vi "FGVScanParametersWaveform.vi"(7 "Enum":T3, 8 "error in":errorcluster, 9 "Parameters In":T1={"fastRoundPts"=32, "slowRoundPts"=8, "fastWaveType"=enum."Rounded", "slowWaveType"=enum."Triangle", "fastWavePts"=1024, "slowWavePts"=1024, "outputRateHz"=800000, "yOffset"=0.0, "xOffset"=0.0, "scanSizeSlow"=0.001, "scanSizeFast"=0.001, "rotation"=0.0, "timePerLine"=0.01, "numLines"=256, "pointsPerLine"=512, "scanEnable"=FALSE, "slowMoveWavePts"=1024, "slowMoveAccelPts"=128, "moveSpeedSec"=0.2, "singleDirectionScan"=FALSE} {"yOffset" min=0.0 max=1.0 format="%#_6p"; "xOffset" format="%.0p"; "scanSizeSlow" min=0.0 max=1.0 format="%#_6pm"; "scanSizeFast" min=0.0 max=1.0 format="%#_6pm"; "rotation" min=0.0 max=1.0 format="%#_6p"; "timePerLine" min=0.0 max=1.0 format="%#_6p"; "pointsPerLine" min=1 max=100 format="%#_6p"}) -> (0 "error out":errorcluster, 1 "Parameters Out":T1={"fastRoundPts"=32, "slowRoundPts"=8, "fastWaveType"=enum."Rounded", "slowWaveType"=enum."Triangle", "fastWavePts"=1024, "slowWavePts"=1024, "outputRateHz"=800000, "yOffset"=0.0, "xOffset"=0.0, "scanSizeSlow"=0.5, "scanSizeFast"=0.5, "rotation"=0.0, "timePerLine"=0.01, "numLines"=256, "pointsPerLine"=512, "scanEnable"=FALSE, "slowMoveWavePts"=1024, "slowMoveAccelPts"=128, "moveSpeedSec"=0.2, "singleDirectionScan"=FALSE} {"yOffset" min=0.0 max=1.0 format="%#_6p"; "xOffset" format="%.0p"; "scanSizeSlow" min=0.0 max=1.0 format="%#_6p"; "scanSizeFast" min=0.0 max=1.0 format="%#_6p"; "rotation" min=0.0 max=1.0 format="%#_6p"; "timePerLine" min=0.0 max=1.0 format="%#_6p"; "pointsPerLine" min=1 max=100 format="%#_6p"})   [LabVIEW 2016]
uses:
  ScanParametersAllTypeDef.ctl
  controls/ScanWaveform.ctl
  controls/Enum.ctl
panel:
  # "scanWaveFormCtl"
  # "slowMoveParameters"
  # "scanCtl"
  # "ioParams"
  # "scanWaveFormCtl"
  # "slowMoveParameters"
  # "scanCtl"
  # "ioParams"
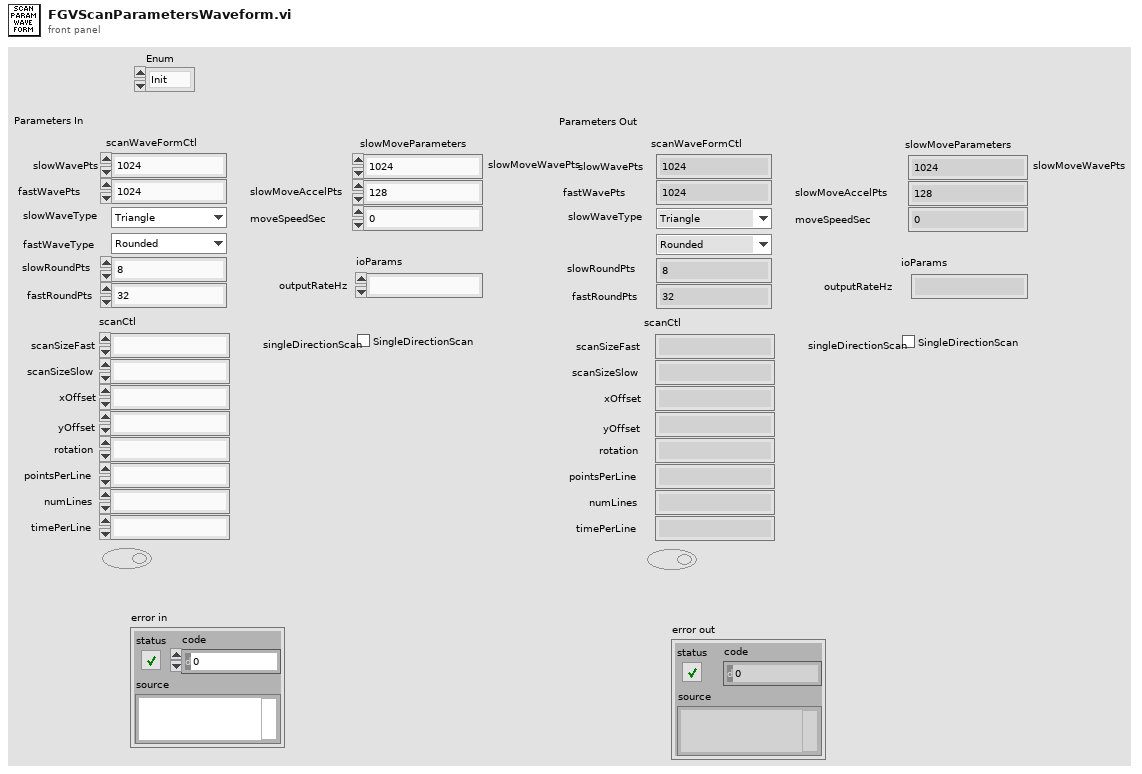
[diagram p1: front panel]
types:
  T1 = typedef "ScanParametersAllTypeDef.ctl" = cluster{"fastRoundPts":u16, "slowRoundPts":u16, "fastWaveType":T2, "slowWaveType":T2, "fastWavePts":u16, "slowWavePts":u16, "outputRateHz":u32, "yOffset":dbl, "xOffset":dbl, "scanSizeSlow":dbl, "scanSizeFast":dbl, "rotation":dbl, "timePerLine":dbl, "numLines":u16, "pointsPerLine":u32, "scanEnable":bool, "slowMoveWavePts":u16, "slowMoveAccelPts":u16, "moveSpeedSec":dbl, "singleDirectionScan":bool}
  T2 = typedef "ScanWaveform.ctl" = enum16{"Sine", "Triangle", "Rounded"}
  T3 = typedef "Enum.ctl" = enum16{"Init", "Read", "Write"}
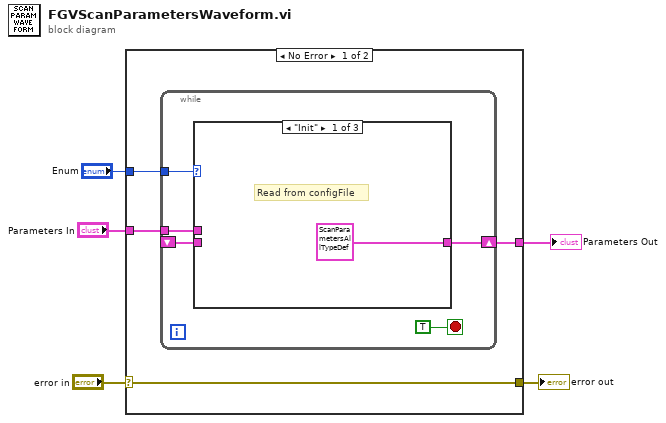
[diagram p0: block diagram]
diagram:
  n1 = case shown="No Error" "error in" {
    selector: "error in" -> [w8 w19]
    tunnel: "Enum" -> [w9 _]
    tunnel: [w8 w19] -> w4
    tunnel: "Parameters In" -> [w7 w18]
    tunnel: [w6 w18] -> w1
    frame No Error {
      n2 = while {
        tunnel: w9 -> [w13]
        tunnel: w7 -> [w12]
        shift-right: [w11] -> w6
        shift-left: _ -> [w10]
        stop <- TRUE stop-if-true
        n3 = case shown="\"Init\"" w13 {
          tunnel: w12 -> [_ _ w17]
          tunnel: [T1 {"fastRoundPts"=32, "slowRoundPts"=8, "fastWaveType"=enum."Rounded", "slowWaveType"=enum."Triangle", "fastWavePts"=1024, "slowWavePts"=1024, "outputRateHz"=800000, "yOffset"=0.0, "xOffset"=0.0, "scanSizeSlow"=5e-07, "scanSizeFast"=5e-07, "rotation"=0.0, "timePerLine"=1.0, "numLines"=256, "pointsPerLine"=256, "scanEnable"=FALSE, "slowMoveWavePts"=1024, "slowMoveAccelPts"=128, "moveSpeedSec"=0.2, "singleDirectionScan"=FALSE} ("Parameters In") w16 w17] -> w11
          tunnel: w10 -> [_ w16 _]
          frame "Init" {
            # "Read from configFile"
          }
          frame "Read", Default {
          }
          frame "Write" {
          }
        }
      }
    }
    frame Error {
    }
  }
  "error out" <- w4
  "Parameters Out" <- w1
